vi "Handle Last Ack Core.vi"(4 "error in (no error)":errorcluster, 6 "Last Ack":refnum<class "Last Ack.lvclass">, 7 "EMS in":refnum<class "EMS.lvclass">) -> (0 "error out":errorcluster, 3 "EMS out":refnum<class "EMS.lvclass">)   [LabVIEW 2018, in "EMS Core.lvlib" / "EMS.lvclass"]
doc: "(<B>Filename</B>: Actor Framework.lvlib:Actor.lvclass:Handle Last Ack Core.vi)\n\nDefines how the caller actor responds to the Last Ack message from a nested actor. The Last Ack message is the final message a nested actor sends to its caller before it shuts down. The message contains information about the final state of the nested actor.\n\nBy default, this method does nothing except return any error the nested actor sent. A descendant class may override this method to define behavior."
uses:
  EMS.lvclass
  <vilib>/ActorFramework/LastAck/Last Ack.lvclass
  EMS.lvclass/EMS.ctl
  EMS Generic Actor/EMS Generic/EMS Generic.lvclass
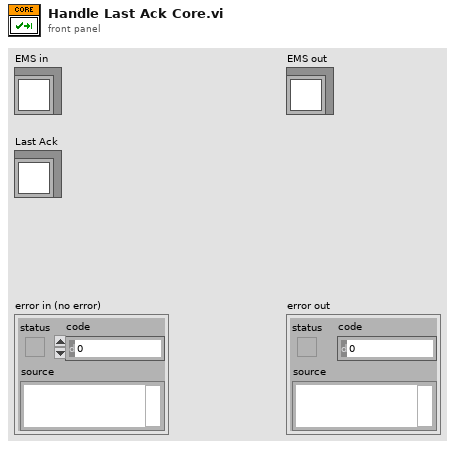
[diagram p1: front panel]
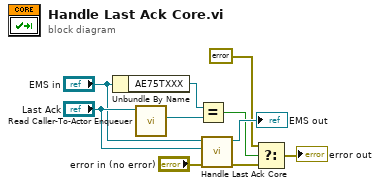
[diagram p0: block diagram]
diagram:
  n1 = Unbundle By Name("EMS in") -> ("AE75TXXX"=w4:refnum<class "Message Enqueuer.lvclass">)
  n2 = call <vilib>:"Read Caller-To-Actor Enqueuer.vi"("Last Ack"="Last Ack") -> ("Caller-to-Actor Enqueuer"=w3:refnum<class "Message Enqueuer.lvclass">)  [unwired: 10 in]
  n3 = Equal?(x=w4, y=w3) -> (x = y?=w2:bool)
  n4 = call-parent "Handle Last Ack Core.vi"("error in (no error)"="error in (no error)", "Last Ack"="Last Ack", "Actor in"="EMS in") -> ("error out"=w7:errorcluster, "Actor out"=→"EMS out":refnum<class "EMS.lvclass">)  [unwired: 3 in]
  n5 = Select(t=errorcluster {"status"=FALSE, "code"=0, "source"=""}, s=w2, f=w7) -> (s? t:f=→"error out":errorcluster)
